vi "Nivel Medido dB.vi"(8 "error in (no error)":errorcluster, 10 "Sensibilidad":dbl(knob)=0.1 scale=0.01..1.0 scale format="%#_6p") -> (0 "error out":errorcluster, 1 "voltaje mV":dbl, 2 "Nivel Medido [dB]":dbl, 3 "AjustesPrevios out":refnum<class "AjustesPrevios.lvclass">)   [LabVIEW 2019, in "AjustesPrevios.lvclass"]
uses:
  AjustesPrevios.lvclass
  Instrumento/Keithley2002/Keithley2002.lvclass
panel:
  out "VAC":string
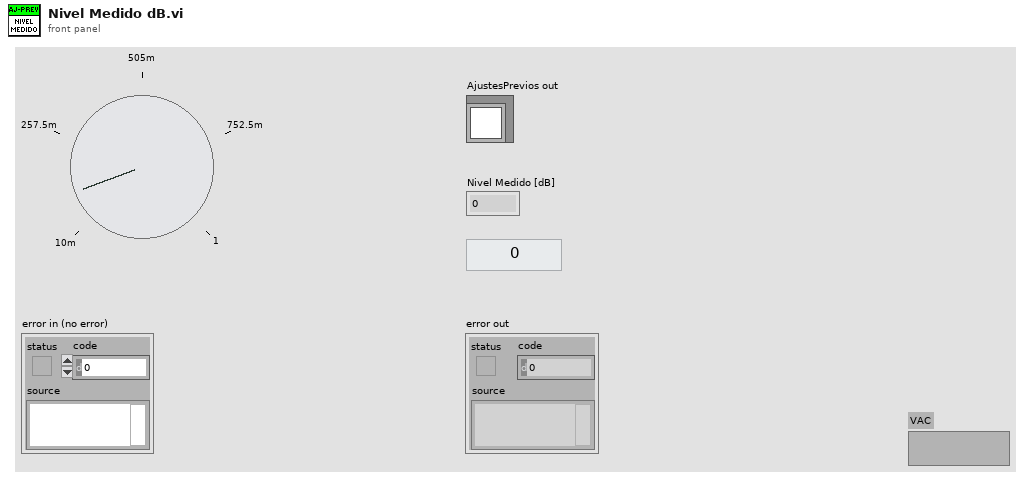
[diagram p1: front panel]
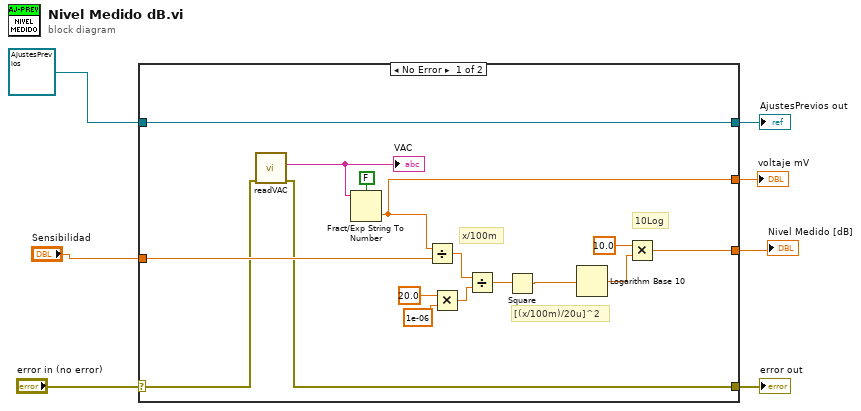
[diagram p0: block diagram]
diagram:
  n1 = case shown="No Error" "error in (no error)" {
    selector: "error in (no error)" -> [w9 w25]
    tunnel: [w8 w25] -> w6
    tunnel: [w23 w24] -> w4
    tunnel: refnum<class "AjustesPrevios.lvclass"> refnum ("AjustesPrevios in") -> [w23 w24]
    tunnel: [w12 _] -> w3
    tunnel: "Sensibilidad" -> [w11 _]
    tunnel: [w10 _] -> w1
    frame No Error {
      # "10Log"
      # "[(x/100m)/20u]^2"
      # "x/100m"
      n2 = call "readVAC.vi"("error in (no error)"=w9) -> ("error out"=w8:errorcluster, "Reading Result"=w21:string)  [unwired: 7 in, 2 out]
      "VAC" <- w21
      n3 = Fract/Exp String To Number(use system decimal point (T)=FALSE, string=w21) -> (number=w10:dbl)  [unwired: 2 in, 1 out]
      n4 = Divide(x=w10, y=w11) -> (x/y=w20:dbl)
      n5 = Multiply(x=20.0, y=1e-06) -> (x*y=w17:dbl)
      n6 = Divide(x=w20, y=w17) -> (x/y=w16:dbl)
      n7 = Square(x=w16) -> (x^2=w13:dbl)
      n8 = Logarithm Base 10(1:w13) -> (0:w14:dbl)
      n9 = Multiply(x=10.0, y=w14) -> (x*y=w12:dbl)
    }
    frame Error {
    }
  }
  "error out" <- w6
  "AjustesPrevios out" <- w4
  "Nivel Medido [dB]" <- w3
  "voltaje mV" <- w1
